vi "ClassPanel.vi"(8 "error in (no error)":errorcluster caption="entrée d'erreur (pas d'erreur)", 11 "YokoGS200.lvclass":refnum<class "YokoGS200.lvclass">) -> (0 "error out":errorcluster caption="sortie d'erreur", 3 "YokoGS200.lvclass Out":refnum<class "YokoGS200.lvclass">)   [LabVIEW 2019, in "YokoGS200.lvclass"]
uses:
  YokoGS200.lvclass
  C:/Programmes Labview/LabScanV1A/DevicesClass/BaseDevice/BaseDevice.lvclass
  BaseDevice/Accessor/GetClassEvent.vi
panel:
  in  "Rate":dbl=1e-06 caption="Ramp Rate(Unit/s)" min=1e-06 step=1e-06
  in  "Ramp":bool=TRUE
  in  "Auto Range":bool
  in  "CurrLim":dbl=0.001 caption="Current Limit" min=0.001 max=0.2 step=0.001
  in  "VoltLim":dbl=1.0 caption="Voltage Limit" min=1.0 max=30.0 step=1.0
  in  "SrcRng":T1(ring) caption="Source Range"
  in  "OutState":bool caption="Output State"
  in  "OutLvl":dbl caption="Output Level"
  in  "SrcFunc":enum16{"Current", "Voltage"}(ring) caption="Source Function"
  in  "Stop":bool
  in  "MiseAJour":bool
  out "Init Program":bool
  # "this MUST labeled with class name"
  # "this MUST be present and labeled \"Stop\""
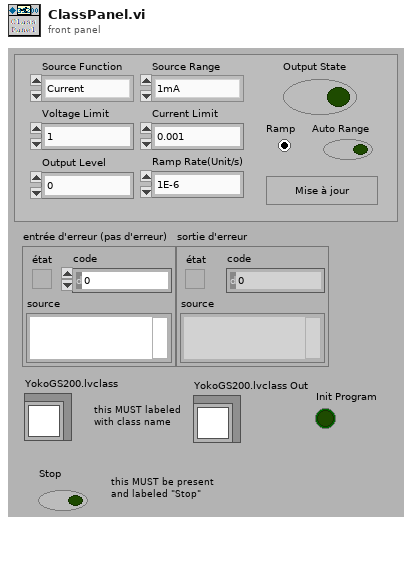
[diagram p1: front panel]
types:
  T1 = enum16{"1mA", "10mA", "100mA", "200mA", "10mV", "100mV", "1V", "10V", "30V", "Minimum", "Maximum"}
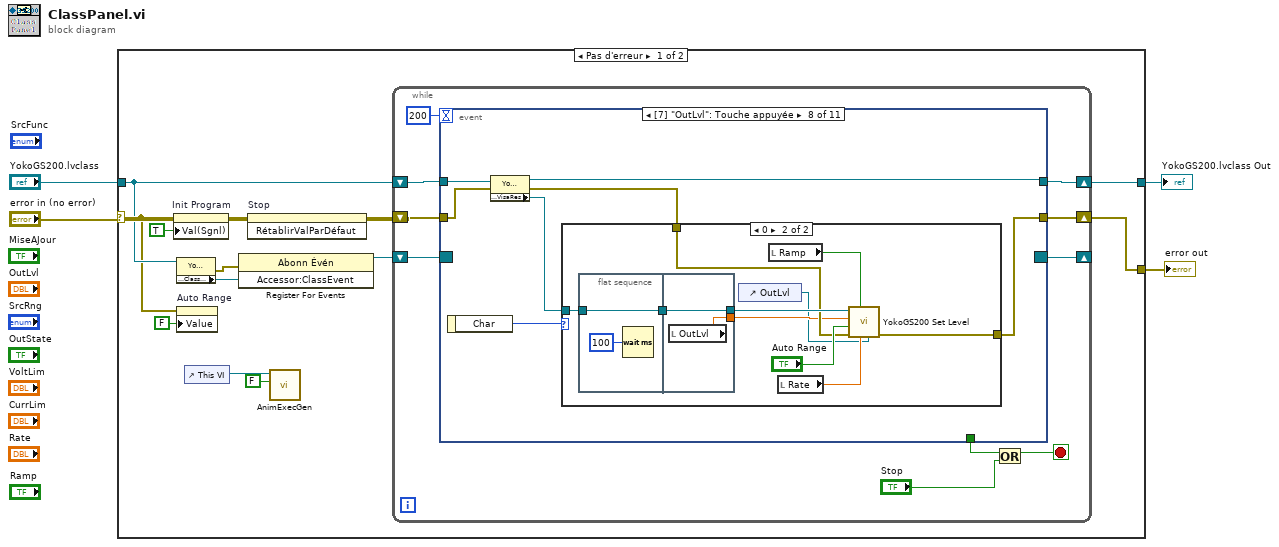
[diagram p0: block diagram]
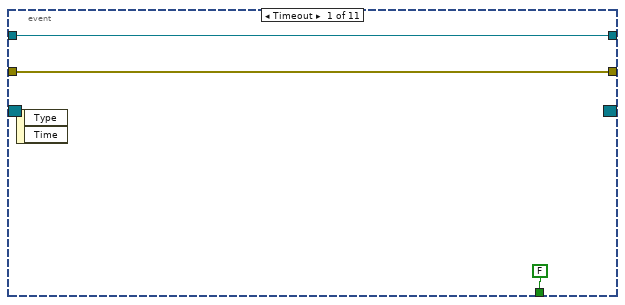
[diagram p2: hidden frame]
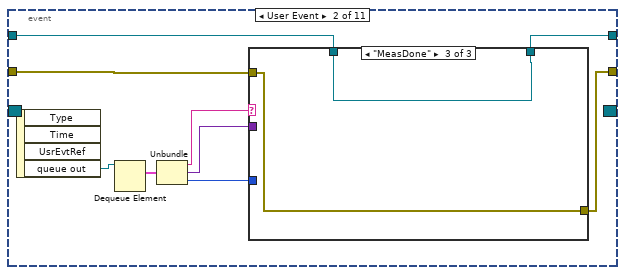
[diagram p3: hidden frame]
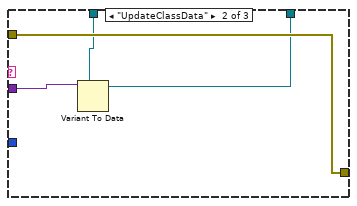
[diagram p5: hidden frame]
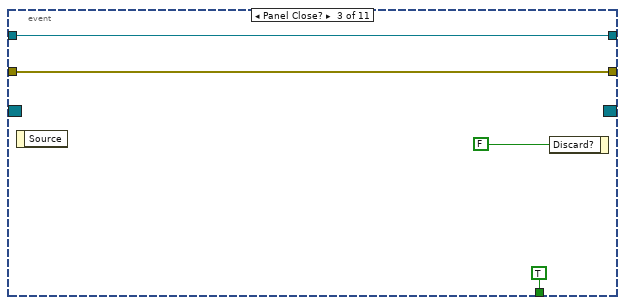
[diagram p6: hidden frame]
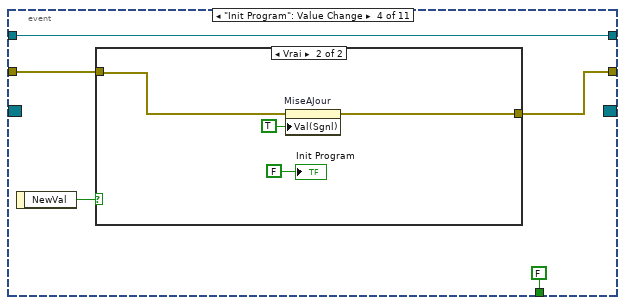
[diagram p7: hidden frame]
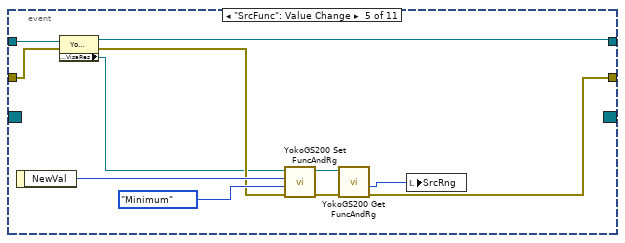
[diagram p9: hidden frame]
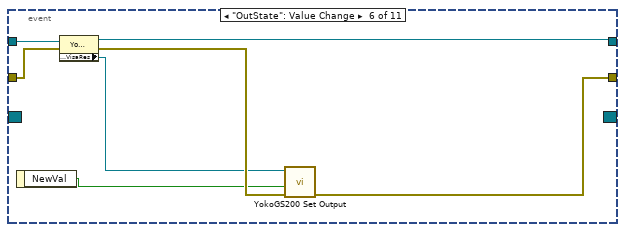
[diagram p10: hidden frame]
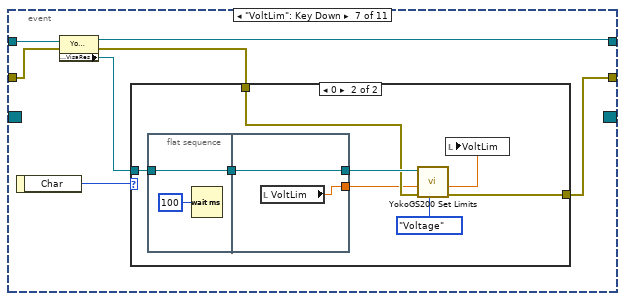
[diagram p11: hidden frame]
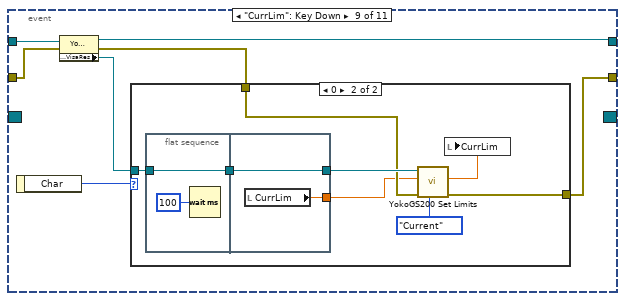
[diagram p14: hidden frame]
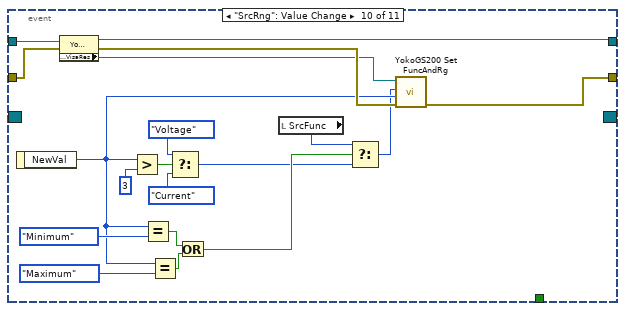
[diagram p16: hidden frame]
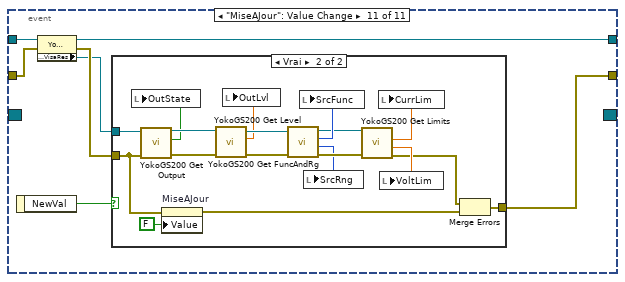
[diagram p17: hidden frame]
diagram:
  n1 = case shown="Pas d'erreur" "error in (no error)" {
    selector: "error in (no error)" -> [w5 w188]
    tunnel: [w17 w188] -> w3
    tunnel: "YokoGS200.lvclass" -> [w10 w187]
    tunnel: [w15 w187] -> w1
    frame No Error {
      n2 = property on="Init Program" class="Bool (strict)"(error in=w5, "Val(Sgnl)"=TRUE ("Valeur (Signalisation)")) -> (error out=w14:errorcluster)  [unwired: 1 in, 1 out]
      n3 = property class="YokoGS200.lvclass"(reference=w10) -> (error out=w12:errorcluster, "Accessor:ClassEvent"=w11:refnum<user-event>)  [unwired: 1 in, 1 out]
      n4 = property on="Auto Range" class="Bool (strict)"(error in=w5, "Value"=FALSE ("Auto Range")) -> ()  [unwired: 1 in, 2 out]
      n5 = control-ref of="This VI"() -> (w7:refnum<vi>)
      n6 = register-events(error in=w12, w11) -> (reference out=w9:refnum<event-registration>)  [unwired: 1 in, 1 out]
      n7 = invoke on="Stop" class="Bool (strict)" method="RétablirValParDéfaut"(error in=w14) -> (error out=w13:errorcluster)  [unwired: 2 in, 2 out]
      n8 = call <userlib>:"AnimExecGen.vi"("Animer l'exécution ?"=FALSE, "ViRef"=w7) -> ()  [unwired: 9 in, 1 out]
      n9 = while {
        shift-right: [w25] -> w17
        shift-left: w13 -> [w26]
        shift-right: [w22] -> w15
        shift-left: w10 -> [w24]
        shift-right: [w18] -> _
        shift-left: w9 -> [w19]
        stop <- w21 stop-if-true
        n10 = event shown="[7] \"OutLvl\": Touche appuyée" {
          selector: w19 -> [_ _ _ _ _ _ _ _ _ _ _]
          dyn-events: [_ _ _ _ _ _ _ _ _ _ _] -> w18
          timeout: 200 -> [_ _ _ _ _ _ _ _ _ _ _]
          tunnel: w26 -> [w28 w38 w49 w55 w68 w77 w84 w104 w126 w158 w165]
          tunnel: [w28 w32 w49 w54 w63 w74 w81 w101 w123 w155 w161] -> w25
          tunnel: w24 -> [w29 w39 w48 w53 w70 w79 w86 w106 w128 w160 w166]
          tunnel: [FALSE _ TRUE FALSE _ _ _ _ _ _ _] -> w23
          tunnel: [w29 w31 w48 w53 w69 w78 w85 w105 w127 w159 w162] -> w22
          event Timeout {
            n11 = event-data() -> ()  [unwired: 1 in, 2 out]
          }
          event User Event {
            n12 = event-data() -> ("queue out"=w36:refnum<queue>)  [unwired: 1 in, 3 out]
            n13 = Dequeue Element(queue=w36) -> (element=w37:cluster{"Message":string, "Data":variant, i32})  [unwired: 2 in, 3 out]
            n14 = Unbundle(w37) -> ("Message"=w35:string, "Data"=w34:variant, w33:i32)
            n15 = case shown="\"MeasDone\"" w35 {
              tunnel: w38 -> [w41 w45 w46]
              tunnel: w34 -> [_ w44 _]
              tunnel: w39 -> [w40 w43 w47]
              tunnel: [w40 w42 w47] -> w31
              tunnel: [w41 w45 w46] -> w32
              tunnel: w33 -> [_ _ _]
              frame Default {
              }
              frame "UpdateClassData" {
                n16 = Variant To Data(type=w43, Variant=w44) -> (data=w42:refnum<class "YokoGS200.lvclass">)  [unwired: 1 in, 1 out]
              }
              frame "MeasDone" {
              }
            }
          }
          event Panel Close? {
            n17 = event-data() -> ()  [unwired: 1 in, 1 out]
            n18 = event-data("Discard?"=FALSE ("Rejeter ?")) -> ()  [unwired: 1 in, 1 out]
          }
          event "Init Program": Value Change {
            n19 = event-data() -> ("NewVal"=w56:bool)  [unwired: 1 in]
            n20 = case shown="Vrai" w56 {
              tunnel: w55 -> [w57 w58]
              tunnel: [w57 w60] -> w54
              frame False {
              }
              frame True {
                n21 = property on="MiseAJour" class="Bool (strict)"(error in=w58, "Val(Sgnl)"=TRUE ("Value (Signaling)")) -> (error out=w60:errorcluster)  [unwired: 1 in, 1 out]
                "Init Program" <- FALSE
              }
            }
          }
          event "SrcFunc": Value Change {
            n22 = event-data() -> ("NewVal"=w72:enum16{"Current", "Voltage"})  [unwired: 1 in]
            n23 = property class="YokoGS200.lvclass"(reference=w70, error in=w68) -> (reference out=w69:refnum<class "YokoGS200.lvclass">, error out=w67:errorcluster, "Accessor:VisaRes"=w66:refnum<visa-resource-name>)
            n24 = call <userlib>:"YokoGS200 Set FuncAndRg.vi"("error in (no error)"=w67, "Source Range"=T1."Minimum", "Source Function"=w72, "VISA Rsrc"=w66) -> ("error out"=w64:errorcluster, "VISA Rsrc Out"=w65:refnum<visa-resource-name>)  [unwired: 5 in, 1 out]
            n25 = call <userlib>:"YokoGS200 Get FuncAndRg.vi"("error in (no error)"=w64, "VISA Rsrc"=w65) -> ("error out"=w63:errorcluster, "Source Range"=w62:T1)  [unwired: 5 in, 3 out]
            n26 = local write "SrcRng"(w62) -> ()
          }
          event "OutState": Value Change {
            n27 = event-data() -> ("NewVal"=w73:bool)  [unwired: 1 in]
            n28 = property class="YokoGS200.lvclass"(reference=w79, error in=w77) -> (reference out=w78:refnum<class "YokoGS200.lvclass">, error out=w76:errorcluster, "Accessor:VisaRes"=w75:refnum<visa-resource-name>)
            n29 = call <userlib>:"YokoGS200 Set Output.vi"("error in (no error)"=w76, "Output State"=w73, "VISA Rsrc"=w75) -> ("error out"=w74:errorcluster)  [unwired: 7 in, 1 out]
          }
          event "VoltLim": Key Down {
            n30 = event-data() -> ("Char"=w80:i16)  [unwired: 1 in]
            n31 = property class="YokoGS200.lvclass"(reference=w86, error in=w84) -> (reference out=w85:refnum<class "YokoGS200.lvclass">, error out=w83:errorcluster, "Accessor:VisaRes"=w82:refnum<visa-resource-name>)
            n32 = case shown="0" w80 {
              tunnel: w83 -> [w87 w90]
              tunnel: w82 -> [_ w92]
              tunnel: [w87 w95] -> w81
              frame Default {
              }
              frame 0 {
                n33 = flat-sequence {
                  tunnel: w92 -> [w96]
                  tunnel: [w96] -> w89
                  tunnel: [w99] -> w91
                  tunnel: w89 -> [w99]
                  tunnel: [w98] -> w88
                  frame #0 {
                    n34 = Wait (ms)(milliseconds to wait=u32 100) -> ()  [unwired: 1 out]
                  }
                  frame #1 {
                    n35 = local read "VoltLim"() -> (w98:dbl)
                  }
                }
                n36 = call <userlib>:"YokoGS200 Set Limits.vi"("Set Limit"=enum16{"Current", "Voltage", "Both"}."Voltage", "error in (no error)"=w90, "VoltLimit"=w88, "VISA Rsrc"=w91) -> ("error out"=w95:errorcluster, "VoltLimit 2"=w93:dbl)  [unwired: 3 in, 3 out]
                n37 = local write "VoltLim"(w93) -> ()
              }
            }
          }
          event "OutLvl": Key Down {
            n38 = event-data() -> ("Char"=w100:i16)  [unwired: 1 in]
            n39 = property class="YokoGS200.lvclass"(reference=w106, error in=w104) -> (reference out=w105:refnum<class "YokoGS200.lvclass">, error out=w103:errorcluster, "Accessor:VisaRes"=w102:refnum<visa-resource-name>)
            n40 = case shown="0" w100 {
              tunnel: w103 -> [w107 w113]
              tunnel: w102 -> [_ w116]
              tunnel: [w107 w117] -> w101
              frame Default {
              }
              frame 0 {
                n41 = flat-sequence {
                  tunnel: w116 -> [w118]
                  tunnel: [w118] -> w112
                  tunnel: [w121] -> w115
                  tunnel: w112 -> [w121]
                  tunnel: [w120] -> w111
                  frame #0 {
                    n42 = Wait (ms)(milliseconds to wait=u32 100) -> ()  [unwired: 1 out]
                  }
                  frame #1 {
                    n43 = local read "OutLvl"() -> (w120:dbl)
                  }
                }
                n44 = control-ref of="OutLvl"() -> (w109:refnum<vi>)
                n45 = local read "Ramp"() -> (w108:bool)
                n46 = local read "Rate"() -> (w110:dbl)
                n47 = call <userlib>:"YokoGS200 Set Level.vi"("CtrlRef"=w109, "RampRate(Unit/s)"=w110, "Ramp"=w108, "error in (no error)"=w113, "Auto Range"="Auto Range", "Output Level"=w111, "VISA Rsrc"=w115) -> ("error out"=w117:errorcluster)  [unwired: 3 in, 1 out]
              }
            }
          }
          event "CurrLim": Key Down {
            n48 = event-data() -> ("Char"=w122:i16)  [unwired: 1 in]
            n49 = property class="YokoGS200.lvclass"(reference=w128, error in=w126) -> (reference out=w127:refnum<class "YokoGS200.lvclass">, error out=w125:errorcluster, "Accessor:VisaRes"=w124:refnum<visa-resource-name>)
            n50 = case shown="0" w122 {
              tunnel: w125 -> [w129 w131]
              tunnel: w124 -> [_ w133]
              tunnel: [w129 w137] -> w123
              frame Default {
              }
              frame 0 {
                n51 = flat-sequence {
                  tunnel: w133 -> [w138]
                  tunnel: [w138] -> w132
                  tunnel: [w141] -> w134
                  tunnel: w132 -> [w141]
                  tunnel: [w140] -> w130
                  frame #0 {
                    n52 = Wait (ms)(milliseconds to wait=u32 100) -> ()  [unwired: 1 out]
                  }
                  frame #1 {
                    n53 = local read "CurrLim"() -> (w140:dbl)
                  }
                }
                n54 = call <userlib>:"YokoGS200 Set Limits.vi"("Set Limit"=enum16{"Current", "Voltage", "Both"}."Current", "error in (no error)"=w131, "CurrLimit"=w130, "VISA Rsrc"=w134) -> ("error out"=w137:errorcluster, "CurrLimit Out"=w135:dbl)  [unwired: 3 in, 3 out]
                n55 = local write "CurrLim"(w135) -> ()
              }
            }
          }
          event "SrcRng": Value Change {
            n56 = event-data() -> ("NewVal"=w149:T1)  [unwired: 1 in]
            n57 = property class="YokoGS200.lvclass"(reference=w160, error in=w158) -> (reference out=w159:refnum<class "YokoGS200.lvclass">, error out=w157:errorcluster, "Accessor:VisaRes"=w156:refnum<visa-resource-name>)
            n58 = Greater?(x=w149, y=3) -> (0:w145:bool)
            n59 = Equal?(x=w149, y=T1."Minimum") -> (x = y?=w152:bool)
            n60 = Equal?(x=w149, y=T1."Maximum") -> (x = y?=w153:bool)
            n61 = Select(t=enum16{"Current", "Voltage"}."Voltage" ("SrcFunc"), s=w145, f=enum16{"Current", "Voltage"}."Current" ("SrcFunc")) -> (s? t:f=w142:enum16{"Current", "Voltage"})
            n62 = Or(x=w152, y=w153) -> (x .or. y?=w148:bool)
            n63 = local read "SrcFunc"() -> (w147:enum16{"Current", "Voltage"})
            n64 = Select(t=w147, s=w148, f=w142) -> (s? t:f=w146:enum16{"Current", "Voltage"})
            n65 = call <userlib>:"YokoGS200 Set FuncAndRg.vi"("error in (no error)"=w157, "Source Range"=w149, "Source Function"=w146, "VISA Rsrc"=w156) -> ("error out"=w155:errorcluster)  [unwired: 5 in, 2 out]
          }
          event "MiseAJour": Value Change {
            n66 = event-data() -> ("NewVal"=w167:bool)  [unwired: 1 in]
            n67 = property class="YokoGS200.lvclass"(reference=w166, error in=w165) -> (reference out=w162:refnum<class "YokoGS200.lvclass">, error out=w164:errorcluster, "Accessor:VisaRes"=w163:refnum<visa-resource-name>)
            n68 = case shown="Vrai" w167 {
              tunnel: w164 -> [w168 w176]
              tunnel: w163 -> [_ w181]
              tunnel: [w168 w169] -> w161
              frame False {
              }
              frame True {
                n69 = call <userlib>:"YokoGS200 Get Output.vi"("VISA Rsrc"=w181, "error in (no error)"=w176) -> ("VISA Rsrc Out"=w182:refnum<visa-resource-name>, "Output State"=w178:bool, "error out"=w183:errorcluster)  [unwired: 6 in]
                n70 = local write "OutState"(w178) -> ()
                n71 = property on="MiseAJour" class="Bool (strict)"(error in=w176, "Value"=FALSE ("MiseAJour")) -> (error out=w171:errorcluster)  [unwired: 1 in, 1 out]
                n72 = call <userlib>:"YokoGS200 Get Level.vi"("VISA Rsrc"=w182, "error in (no error)"=w183) -> ("VISA Rsrc Out"=w184:refnum<visa-resource-name>, "Output Level"=w180:dbl, "error out"=w185:errorcluster)  [unwired: 6 in]
                n73 = local write "OutLvl"(w180) -> ()
                n74 = call <userlib>:"YokoGS200 Get FuncAndRg.vi"("error in (no error)"=w185, "VISA Rsrc"=w184) -> ("error out"=w175:errorcluster, "Source Range"=w174:T1, "Source Function"=w179:enum16{"Current", "Voltage"}, "VISA Rsrc Out"=w177:refnum<visa-resource-name>)  [unwired: 5 in, 1 out]
                n75 = local write "SrcFunc"(w179) -> ()
                n76 = local write "SrcRng"(w174) -> ()
                n77 = call <userlib>:"YokoGS200 Get Limits.vi"("error in (no error)"=w175, "VISA Rsrc"=w177) -> ("error out"=w172:errorcluster, "VoltLimit"=w173:dbl, "CurrLimit"=w170:dbl)  [unwired: 6 in, 1 out]
                n78 = local write "CurrLim"(w170) -> ()
                n79 = local write "VoltLim"(w173) -> ()
                n80 = Merge Errors(w172, w171) -> (w169:errorcluster)
              }
            }
          }
        }
        n81 = Or(x=w23, y="Stop") -> (x .or. y?=w21:bool)
      }
    }
    frame Error {
    }
  }
  "error out" <- w3
  "YokoGS200.lvclass Out" <- w1
